vi "Configure Channel Unit.vi"(8 "error in (no error)":errorcluster, 9 "Unit (0: Volts)":u16(ring) items=["Volts", "Amperes", "Watts", "Unknown"], 10 "Channel Name (0: Channel 1)":u16(ring) items=["Channel 1", "Channel 2", "Channel 3", "Channel 4"], 11 "VISA resource name":refnum<visa-resource-name>) -> (0 "error out":errorcluster, 3 "VISA resource name out":refnum<visa-resource-name>)   [LabVIEW 2025, in "RIGOL MHO900 Series.lvlib"]
uses:
  RIGOL MHO900 Series.lvlib
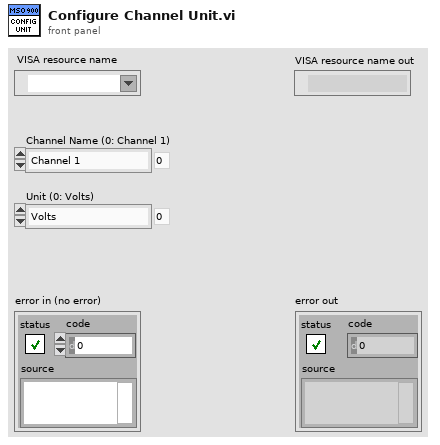
[diagram p1: front panel]
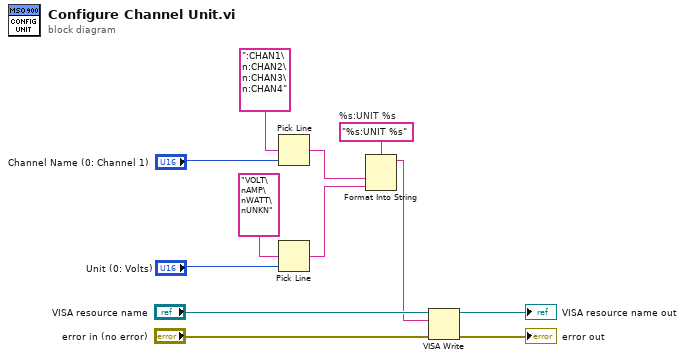
[diagram p0: block diagram]
diagram:
  w10 = "%s:UNIT %s"  # %s:UNIT %s
  n1 = Pick Line(multi-line string=":CHAN1\n:CHAN2\n:CHAN3\n:CHAN4", line index="Channel Name (0: Channel 1)") -> (output string=w5:string)  [unwired: 1 out]
  n2 = Pick Line(multi-line string="VOLT\nAMP\nWATT\nUNKN", line index="Unit (0: Volts)") -> (output string=w2:string)  [unwired: 1 out]
  n3 = Format Into String(format string=w10, w5, w2) -> (resulting string=w9:string)  [unwired: 2 in, 1 out]
  n4 = VISA Write(VISA resource name="VISA resource name", write buffer=w9, error in (no error)="error in (no error)") -> (VISA resource name out=→"VISA resource name out":refnum<visa-resource-name>, error out=→"error out":errorcluster)  [unwired: 1 out]
